vi "client.vi"() -> ()   [LabVIEW 2020]
uses:
  16ec9fc5-b449-4fd0-8ebf-c19c0618ca31.vi
  <vilib>/Utility/file.llb/Write Delimited Spreadsheet (string).vi
panel:
  in  "file path (dialog if empty)":path
  in  "stop":bool
  in  "Tamper":bool
  in  "Alarm":bool
  in  "Bypass":bool
  # "Zone 1"
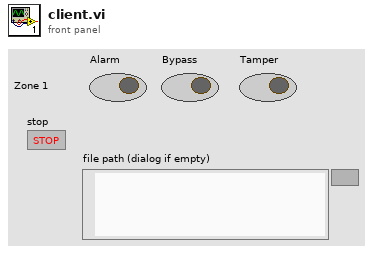
[diagram p1: front panel]
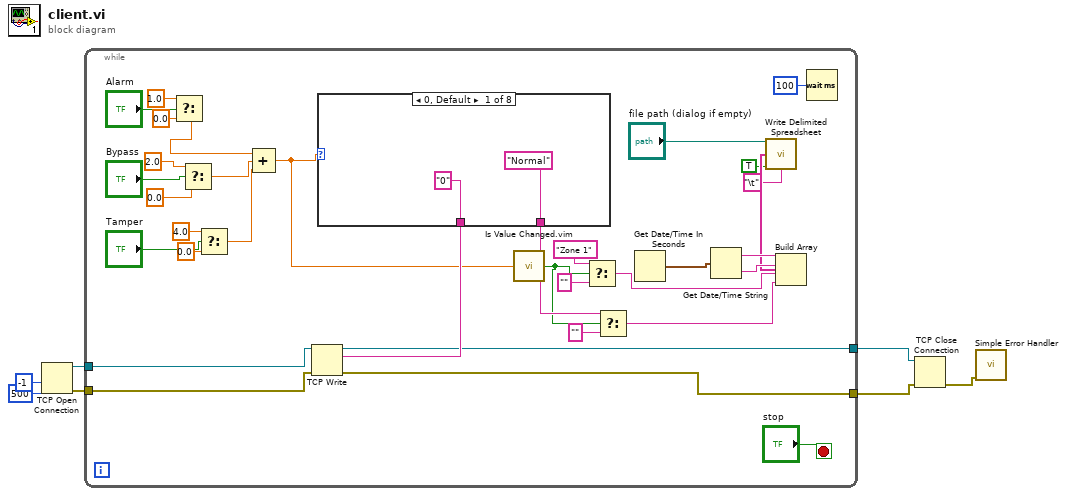
[diagram p0: block diagram]
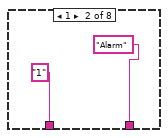
[diagram p2: hidden frame]
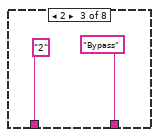
[diagram p3: hidden frame]
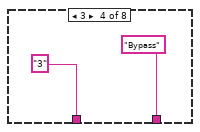
[diagram p4: hidden frame]
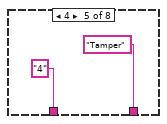
[diagram p5: hidden frame]
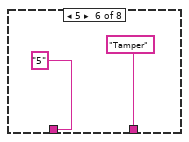
[diagram p6: hidden frame]
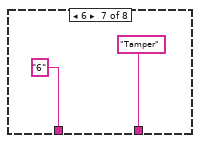
[diagram p7: hidden frame]
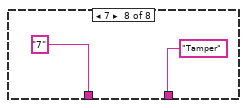
[diagram p8: hidden frame]
diagram:
  n1 = TCP Open Connection(remote port or service name=u16 500, timeout ms (60000)=-1) -> (connection ID=w7:refnum<k5>, error out=w6:errorcluster)  [unwired: 3 in]
  n2 = while {
    tunnel: w7 -> [w28]
    tunnel: w6 -> [w27]
    tunnel: [w26] -> w5
    tunnel: [w23] -> w1
    stop <- "stop" stop-if-true
    n3 = Select(t=1.0, s="Alarm", f=0.0) -> (s? t:f=w41:dbl)
    n4 = Select(t=2.0, s="Bypass", f=0.0) -> (s? t:f=w34:dbl)
    n5 = Select(t=4.0, s="Tamper", f=0.0) -> (s? t:f=w30:dbl)
    n6 = Compound Arithmetic op=ADD(w41, w34, w30) -> (w18:dbl)
    n7 = case shown="0, Default" w18 {
      tunnel: ["0" "1" "2" "3" "4" "5" "6" "7"] -> w25
      tunnel: ["Normal" "Alarm" "Bypass" "Bypass" "Tamper" "Tamper" "Tamper" "Tamper"] -> w14
      frame 0, Default {
      }
      frame 1 {
      }
      frame 2 {
      }
      frame 3 {
      }
      frame 4 {
      }
      frame 5 {
      }
      frame 6 {
      }
      frame 7 {
      }
    }
    n8 = TCP Write(connection ID=w28, data in=w25, error in (no error)=w27) -> (connection ID out=w23:refnum<k5>, error out=w26:errorcluster)  [unwired: 1 in, 1 out]
    n9 = call "Is Value Changed.vim"("value"=w18) -> ("changed or first call?"=w13:bool)
    n10 = Select(t="Zone 1", s=w13, f="") -> (s? t:f=w15:string)
    n11 = Select(t=w14, s=w13, f="") -> (s? t:f=w11:string)
    n12 = Get Date/Time In Seconds() -> (seconds since 1Jan1904=w21:timestamp)
    n13 = Get Date/Time String(seconds (now)=w21) -> (date string=w20:string, time string=w19:string)  [unwired: 2 in]
    n14 = Build Array(w20, w19, w15, w11) -> (w10:string[])
    n15 = call-poly <vilib>:"Write Delimited Spreadsheet.vi"("file path (dialog if empty)"="file path (dialog if empty)", "1D data"=w10, "append to file? (new file:F)"=TRUE, "delimiter (\\t)"="\t" ("delimiter (\\t)")) -> ()  [unwired: 10 in, 2 out]
    n16 = Wait (ms)(milliseconds to wait=u32 100) -> ()  [unwired: 1 out]
  }
  n17 = TCP Close Connection(connection ID=w1, error in (no error)=w5) -> (error out=w2:errorcluster)  [unwired: 1 in, 1 out]
  n18 = call <vilib>:"Simple Error Handler.vi"("error in (no error)"=w2) -> ()  [unwired: 4 in, 5 out]
